vi "Dashboard Main.vi"() -> ()   [LabVIEW 2011]
uses:
  subStates.ctl
  <vilib>/Rock Robotics/WPI/DriverStation/WPI_DriverStationDigitalData.ctl
  <userlib>/_MGI/1D Array/MGI Running Minimum/MGI Running Minimum (SGL).vi
  <userlib>/_MGI/1D Array/MGI Running Maximum/MGI Running Maximum (SGL).vi
  <userlib>/_MGI/1D Array/MGI Running Average/MGI Running Average(SGL).vi
panel:
  in  "Target Overlay":bool=TRUE
  in  "Video Enable":bool=TRUE
  out "Camera Image":T1(plugin-control)
  in  "Info Tabz":enum32{"Comp", "Debug", "UberDebug", "Stats"}(tab)
  out "Shooter Bias":dbl(slide) caption="SHOOTER BIAS" scale=-0.2..0.2
  out "TURRET SAFETY":bool
  out "TURRET LIMIT":bool
  out "GEAR":bool
  out "TRACKING":bool
  out "HOLD":bool
  out "VLAD":bool
  out "Shooter Speed Comp":dbl(slide) caption="SHOOTER SPEED" scale=0.0..100.0
  out "Rest of Custom Data":string
  out "Solenoid Output":bool[](array[boolean])
  out "Robot IP Address":string
  out "8 -- Battery":sgl(graph)
  out "Analog Input":sgl[](array[slide]) scale=0.0..5.0
  out "PWM":cluster{u8, u8}[](array[slide])=[{0, 157}, {0, 157}, {0, 157}, {0, 157}, {0, 157}, {0, 157}, {0, 157}, {0, 157}, {0, 157}, {0, 169}] scale=1.0..255.0
  out "GPIO Output Enable":bool[](array[boolean])
  out "GPIO State":bool[](array[boolean])
  out "Relay":cluster{"Forward":bool[], "Reverse":bool[]}
  out "Shooter Speed":dbl(slide) scale=0.0..100.0 scale format="%#.2g%f"
  out "Safety":bool
  out "Turret Distance":dbl caption="Distance" format="%#_3g"
  out "Turret Rate":dbl caption="Rate" format="%#_3g"
  out "Right Distance":dbl caption="Distance" format="%#_3g"
  out "Right Rate":dbl caption="Rate" format="%#_3g"
  out "Left Distance":dbl caption="Distance" format="%#_3g"
  out "Left Rate":dbl caption="Rate" format="%#_3g"
  out "Angle":dbl(knob) scale=-45.0..45.0 scale format="%#_3g"
  out "Ang. Rate":dbl(knob) scale=-45.0..45.0 scale format="%#_3g"
  out "Lower Belts":T2
  out "Upper Belts":T2
  out "Shooter":T2
  out "Turret":T2
  out "Drive":T2
  out "CPU Usage":dbl(knob) scale=0.0..100.0
  out "RAM Available":u32
  out "Average":dbl
  out "Low":sgl
  out "High":sgl
  out "Battery Voltage":sgl(slide) scale=0.0..15.0
  out "Main IPS":dbl
  out "Vision IPS":dbl
  out "IPS":cluster{dbl, dbl}(knob)={0.0, 16.607957775505273} scale=0.0..60.0
  out "Main mSPI":u32
  out "Vision mSPI":u32
  out "Dashboard Datatype Warning":string="Warning: The Dashboard Datatype used by the robot project and this dashboard do not match.\nSee diagram for more details."
  out "Image Error Message":string="Timeout in Camera Communications"
  # "Solenoid #1"
  # "1"
  # "8"
  # "Communications"
  # "Analog #1"
  # "1"
  # "7"
  # "Digital #1"
  # "1"
  # "10"
  # "1"
  # "14"
  # "1"
  # "8"
  # "Robot States"
  # "Drive Encoders"
  # "Left"
  # "Right"
  # "Turret"
  # "Robot Angle"
  # "Code Speed"
  # "Robot Battery"
  # "cRIO Performance"
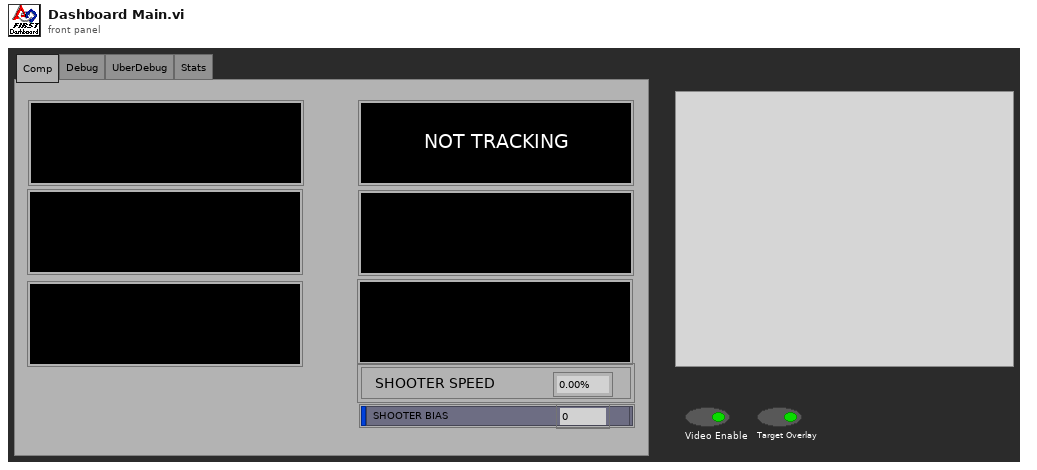
[diagram p1: front panel]
types:
  T1 = typedef "IMAQ Image.ctl" = refnum<image>
  T2 = typedef "subStates.ctl" = enum16{"null", "wait", "driver control", "auto", "manual override", "autoDrive", "hold position", "end"}
  T3 = cluster{"doubles":cluster{"Shooter Speed":dbl, "Turret Rate":dbl, "Turret Distance":dbl, "Right Distance":dbl, "Right Rate":dbl, "Left Rate":dbl, "Left Distance":dbl, "Ang. Rate":dbl, "Angle":dbl, "Shooter Bias":dbl}, "substates":cluster{"Shooter":T2, "Upper Belts":T2, "Lower Belts":T2, "Turret ":T2, "Drive":T2}, "bools":cluster{"VLAD Balanced":bool, "Safety":bool, "Turret Limit":bool}, "Performance":cluster{"CPU Usage":dbl, "RAM Available":u32, "Vision mSPI":u32, "Main mSPI":u32}, "Target Info":cluster{"Left":i32, "Top":i32, "Right":i32, "Bottom":i32}}
  T4 = typedef "WPI_DriverStationDigitalData.ctl" = cluster{"Relay Fwd":u8, "Relay Rev":u8, "GPIO":u16, "GPIO_OE":u16, "PWM":cluster{"PWM[0]":u8, "PWM[1]":u8, "PWM[2]":u8, "PWM[3]":u8, "PWM[4]":u8, "PWM[5]":u8, "PWM[6]":u8, "PWM[7]":u8, "PWM[8]":u8, "PWM[9]":u8}}
  T5 = cluster{cluster{"AnalogModule[0]":cluster{"Channel[0]":sgl, "Channel[1]":sgl, "Channel[2]":sgl, "Channel[3]":sgl, "Channel[4]":sgl, "Channel[5]":sgl, "Channel[6]":sgl, "Channel[7]":sgl}, "AnalogModule[1]":cluster{"Channel[0]":sgl, "Channel[1]":sgl, "Channel[2]":sgl, "Channel[3]":sgl, "Channel[4]":sgl, "Channel[5]":sgl, "Channel[6]":sgl, "Channel[7]":sgl}}, cluster{"DigitalModule[0]":T4, "DigitalModule[1]":T4}, "Solenoid":u8}
  T6 = typedef "Image Type" = u32
  T7 = cluster{"Left":i32, "Top":i32, "Right":i32, "Bottom":i32}
  T8 = cluster{"Competition mode":bool, "Robot Link":bool, "Autonomous":bool, "Enabled":bool, "E-Stop":bool}
  T9 = cluster{"Left":bool, "Top":bool, "Right":bool, "Bottom":bool}
  T10 = cluster{"AnalogModule[0]":cluster{"Channel[0]":sgl, "Channel[1]":sgl, "Channel[2]":sgl, "Channel[3]":sgl, "Channel[4]":sgl, "Channel[5]":sgl, "Channel[6]":sgl, "Channel[7]":sgl}, "AnalogModule[1]":cluster{"Channel[0]":sgl, "Channel[1]":sgl, "Channel[2]":sgl, "Channel[3]":sgl, "Channel[4]":sgl, "Channel[5]":sgl, "Channel[6]":sgl, "Channel[7]":sgl}}
  T11 = cluster{"DigitalModule[0]":T4, "DigitalModule[1]":T4}
  T12 = cluster{"Channel[0]":sgl, "Channel[1]":sgl, "Channel[2]":sgl, "Channel[3]":sgl, "Channel[4]":sgl, "Channel[5]":sgl, "Channel[6]":sgl, "Channel[7]":sgl}[]
  T13 = cluster{"Channel[0]":sgl, "Channel[1]":sgl, "Channel[2]":sgl, "Channel[3]":sgl, "Channel[4]":sgl, "Channel[5]":sgl, "Channel[6]":sgl, "Channel[7]":sgl}
  T14 = typedef "LVRectTypeDef.ctl" = cluster{"left":i16, "top":i16, "right":i16, "bottom":i16}
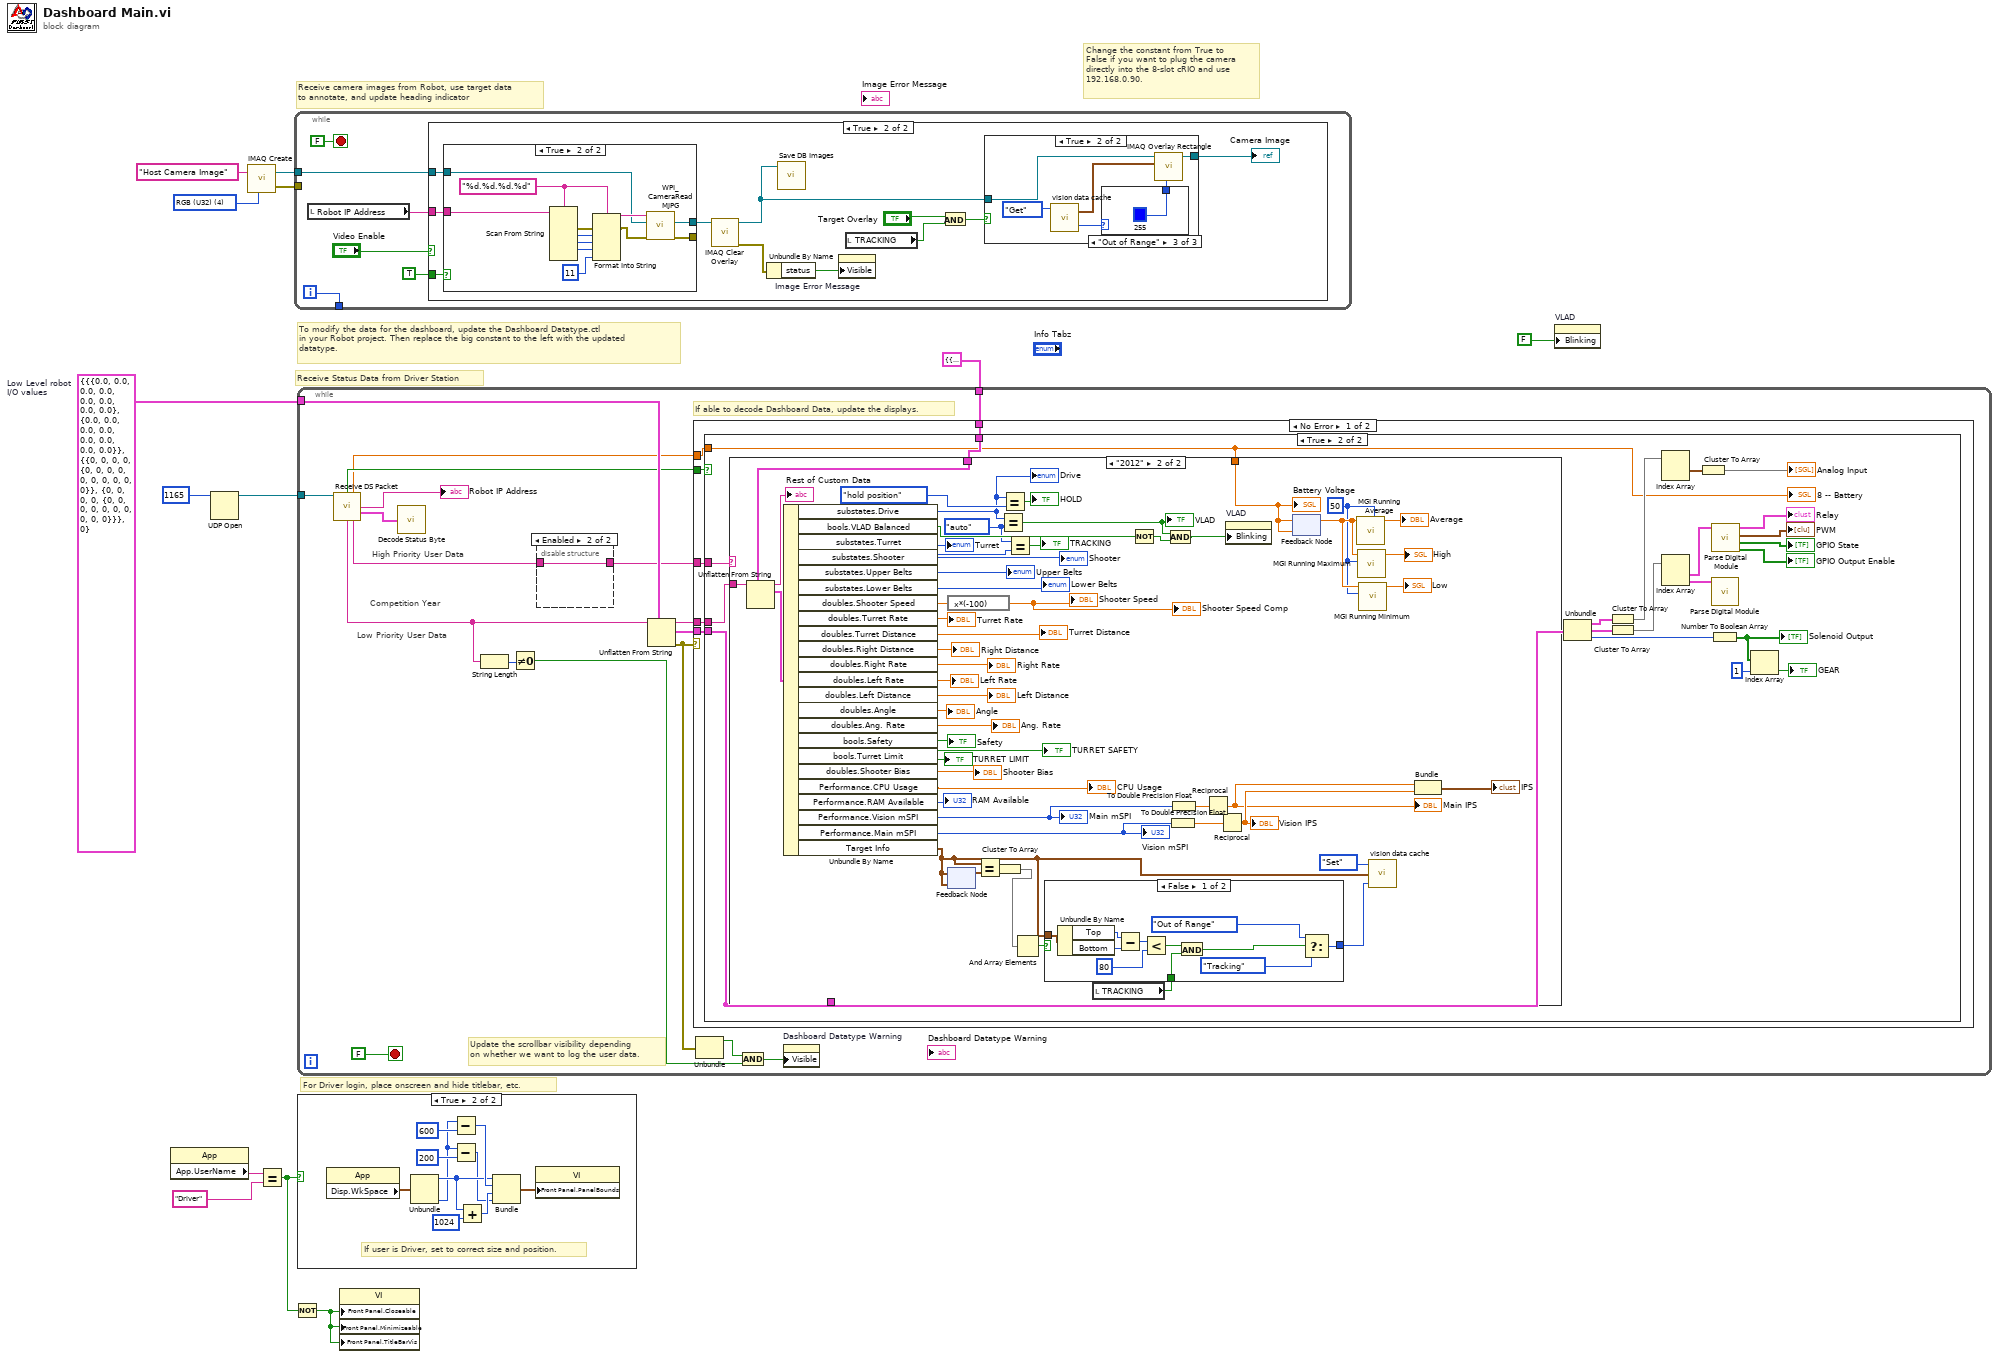
[diagram p0: block diagram]
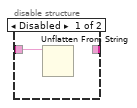
[diagram p3: hidden frame]
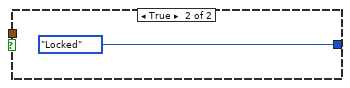
[diagram p6: hidden frame]
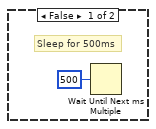
[diagram p8: hidden frame]
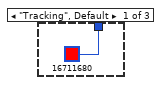
[diagram p10: hidden frame]
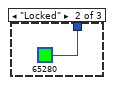
[diagram p11: hidden frame]
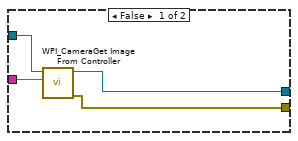
[diagram p12: hidden frame]
diagram:
  w5 = T5 {{"AnalogModule[0]"={"Channel[0]"=0.0, "Channel[1]"=0.0, "Channel[2]"=0.0, "Channel[3]"=0.0, "Channel[4]"=0.0, "Channel[5]"=0.0, "Channel[6]"=0.0, "Channel[7]"=0.0}, "AnalogModule[1]"={"Channel[0]"=0.0, "Channel[1]"=0.0, "Channel[2]"=0.0, "Channel[3]"=0.0, "Channel[4]"=0.0, "Channel[5]"=0.0, "Channel[6]"=0.0, "Channel[7]"=0.0}}, {"DigitalModule[0]"={"Relay Fwd"=0, "Relay Rev"=0, "GPIO"=0, "GPIO_OE"=0, "PWM"={"PWM[0]"=0, "PWM[1]"=0, "PWM[2]"=0, "PWM[3]"=0, "PWM[4]"=0, "PWM[5]"=0, "PWM[6]"=0, "PWM[7]"=0, "PWM[8]"=0, "PWM[9]"=0}}, "DigitalModule[1]"={"Relay Fwd"=0, "Relay Rev"=0, "GPIO"=0, "GPIO_OE"=0, "PWM"={"PWM[0]"=0, "PWM[1]"=0, "PWM[2]"=0, "PWM[3]"=0, "PWM[4]"=0, "PWM[5]"=0, "PWM[6]"=0, "PWM[7]"=0, "PWM[8]"=0, "PWM[9]"=0}}}, "Solenoid"=0}  # Low Level robot I/O values
  w13 = T6 4 items=["Grayscale (U8)", "Grayscale (I16)", "Grayscale (SGL)", "Complex (CSG)", "RGB (U32)", "HSL (U32)", "RGB (U64)"] ("Image Type")
  # "Change the constant from True to\nFalse if you want to plug the camera\ndirectly into the 8-slot cRIO and use\n192.168.0.90."
  # "For Driver login, place onscreen and hide titlebar, etc."
  # "To modify the data for the dashboard, update the Dashboard Datatype.ctl\nin your Robot project. Then replace the big constant to the left with the updated\ndatatype."
  # "Receive Status Data from Driver Station"
  # "Receive camera images from Robot, use target data\nto annotate, and update heading indicator"
  n1 = property class="App"() -> ("App.UserName"=w8:string)  [unwired: 2 in, 2 out]
  n2 = UDP Open(11:u16 1165 ("port")) -> (port=w3:refnum<k16>)  [unwired: 2 in, 4 out]
  n3 = call "IMAQ Create"("Image Name"="Host Camera Image", "Image Type"=w13) -> ("New Image"=w11:T1, "error out"=w10:errorcluster)  [unwired: 2 in, 1 out]
  n4 = Equal?(x=w8, y="Driver") -> (x = y?=w7:bool)
  n5 = Not(x=w7) -> (.not. x?=w6:bool)
  n6 = while {
    tunnel: w11 -> [w17]
    tunnel: w10 -> [_]
    tunnel: [w14] -> _
    i -> [w14]
    stop <- FALSE stop-if-true
    n7 = local read "Robot IP Address"() -> (w18:string)
    n8 = case shown="True" "Video Enable" {
      tunnel: w18 -> [_ w31]
      tunnel: w17 -> [_ w30]
      tunnel: TRUE -> [_ w26]
      frame False {
        # "Sleep for 500ms"
        n9 = Wait Until Next ms Multiple(millisecond multiple=u32 500) -> ()  [unwired: 1 out]
      }
      frame True {
        n10 = case shown="True" w26 {
          tunnel: w30 -> [w44 w51]
          tunnel: [w42 w49] -> _
          tunnel: [w43 w50] -> w27
          tunnel: w31 -> [w45 w54]
          frame False {
            n11 = call <vilib>:"WPI_CameraGet Image From Controller.vi"("Controller Address"=w45, "Image"=w44) -> ("error out"=w42:errorcluster, "Image Out"=w43:T1)  [unwired: 2 in, 6 out]
          }
          frame True {
            w46 = "%d.%d.%d.%d" ("format string")
            n12 = Scan From String(format string=w46, input string=w54) -> (error out=w53:errorcluster, output 1=w55:i32, output 2=w56:i32, output 3=w57:i32)  [unwired: 2 in, 7 out]
            n13 = Format Into String(format string=w46, error in=w53, w55, w56, w57, 11 ("IP Suffix:")) -> (resulting string=w52:string, error out=w48:errorcluster)  [unwired: 1 in]
            n14 = call <vilib>:"WPI_CameraRead MJPG.vi"("error in"=w48, "Image"=w51, "address"=w52) -> ("error out"=w49:errorcluster, "Image Out"=w50:T1)  [unwired: 7 in]
          }
        }
        n15 = call "IMAQ Clear Overlay"("Image"=w27) -> ("error out"=w28:errorcluster, "Image Out"=w25:T1)  [unwired: 2 in, 7 out]
        n16 = Unbundle By Name(w28) -> ("status"=w29:bool)
        n17 = call "Save DB Images.vi"("Image"=w25) -> ()  [unwired: 2 in, 1 out]
        n18 = property on="Image Error Message" class="Str"("Visible"=w29) -> ()  [unwired: 2 in, 2 out]
        n19 = local read "TRACKING"() -> (w22:bool)
        n20 = And(x="Target Overlay", y=w22) -> (x .and. y?=w21:bool)
        n21 = case shown="True" w21 {
          tunnel: w25 -> [w32 w38]
          tunnel: [w32 w35] -> w24
          frame False {
          }
          frame True {
            n22 = call "vision data cache.vi"("Menu (Get)"=enum16{"Get", "Set"}."Get") -> ("State Out"=w34:enum16{"Tracking", "Locked", "Out of Range"}, "Data Output"=w36:T7)  [unwired: 2 in]
            n23 = case shown="\"Out of Range\"" w34 {
              tunnel: [u32 16711680 ("Color") u32 65280 ("Color") u32 255 ("Color")] -> w33
              frame "Tracking", Default {
              }
              frame "Locked" {
              }
              frame "Out of Range" {
              }
            }
            n24 = call "IMAQ Overlay Rectangle"("Color"=w33, "Rectangle"=w36, "Image"=w38) -> ("Image Out"=w35:T1)  [unwired: 3 in, 5 out]
          }
        }
        "Camera Image" <- w24
      }
    }
  }
  n25 = while {
    tunnel: w3 -> [w73]
    tunnel: w5 -> [w72]
    tunnel: T3 {"doubles"={"Shooter Speed"=0.0, "Turret Rate"=0.0, "Turret Distance"=0.0, "Right Distance"=0.0, "Right Rate"=0.0, "Left Rate"=0.0, "Left Distance"=0.0, "Ang. Rate"=0.0, "Angle"=0.0, "Shooter Bias"=0.0}, "substates"={"Shooter"=enum."null", "Upper Belts"=enum."null", "Lower Belts"=enum."null", "Turret "=enum."null", "Drive"=enum."null"}, "bools"={"VLAD Balanced"=FALSE, "Safety"=FALSE, "Turret Limit"=FALSE}, "Performance"={"CPU Usage"=0.0, "RAM Available"=0, "Vision mSPI"=0, "Main mSPI"=0}, "Target Info"={"Left"=0, "Top"=0, "Right"=0, "Bottom"=0}} ("Custom Dash Data") -> [w59]
    stop <- FALSE stop-if-true
    # "Competition Year"
    # "High Priority User Data"
    # "Low Priority User Data"
    # "Update the scrollbar visibility depending\non whether we want to log the user data."
    # "If able to decode Dashboard Data, update the displays."
    n26 = call "Receive DS Packet.vi"("Recv Socket"=w73) -> ("New Dashboard Data"=w69:bool, "Battery"=w60:sgl, "Robot IP Address"=→"Robot IP Address":string, "Status"=w74:T8, "Low Priority User Data"=w62:string, "High Priority User Data"=w61:string)  [unwired: 1 in, 8 out]
    n27 = call "Decode Status Byte.vi"("Status Byte"=w74) -> ()  [unwired: 2 out]
    n28 = String Length(string=w62) -> (length=w64:i32)
    n29 = Not Equal To 0?(x=w64) -> (x != 0?=w67:bool)
    n30 = disable-structure shown="Enabled" {
      disable-tunnel: w61 -> [w76 w77]
      disable-tunnel: [_ w77] -> w58
      frame Disabled {
        n31 = Unflatten From String(binary string=w76) -> ()  [unwired: 2 in, 5 out]
      }
      frame Enabled {
      }
    }
    n32 = Unflatten From String(type=w72, binary string=w62) -> (rest of the binary string=w65:string, value=w71:T5, error out=w70:errorcluster)  [unwired: 1 in, 2 out]
    n33 = case shown="No Error" w70 {
      tunnel: w71 -> [w83 _]
      tunnel: w69 -> [w82 _]
      tunnel: w65 -> [w79 _]
      tunnel: w60 -> [w81 _]
      tunnel: w58 -> [w80 _]
      tunnel: w59 -> [w78 _]
      frame No Error {
        n34 = case shown="True" w82 {
          tunnel: w83 -> [_ w90]
          tunnel: w81 -> [_ w84]
          tunnel: w80 -> [_ w91]
          tunnel: w79 -> [_ w89]
          tunnel: w78 -> [_ w88]
          frame False {
            # "Don't update if the robot hasn't sent new data"
          }
          frame True {
            n35 = case shown="\"2012\"" w91 {
              tunnel: w90 -> [_ _]
              tunnel: w89 -> [_ w156]
              tunnel: w88 -> [_ w157]
              tunnel: w84 -> [_ w121]
              frame "False", Default {
              }
              frame "2012" {
                w117 = 50 ("Averaging Size")
                w114 = subStates."auto" ("y")
                n36 = Unflatten From String(type=w157, binary string=w156) -> (rest of the binary string=→"Rest of Custom Data":string, value=w155:T3)  [unwired: 1 in, 3 out]
                n37 = Unbundle By Name(w155) -> ("substates.Drive"=w136:T2, "bools.VLAD Balanced"=w139:bool, "substates.Turret"=w113:T2, "substates.Shooter"=→"Shooter":T2, "substates.Upper Belts"=→"Upper Belts":T2, "substates.Lower Belts"=→"Lower Belts":T2, "doubles.Shooter Speed"=w150:dbl, "doubles.Turret Rate"=→"Turret Rate":dbl, "doubles.Turret Distance"=→"Turret Distance":dbl, "doubles.Right Distance"=→"Right Distance":dbl, "doubles.Right Rate"=→"Right Rate":dbl, "doubles.Left Rate"=→"Left Rate":dbl, "doubles.Left Distance"=→"Left Distance":dbl, "doubles.Angle"=→"Angle":dbl, "doubles.Ang. Rate"=→"Ang. Rate":dbl, "bools.Safety"=→"Safety" →"TURRET SAFETY":bool, "bools.Turret Limit"=→"TURRET LIMIT":bool, "doubles.Shooter Bias"=→"Shooter Bias":dbl, "Performance.CPU Usage"=→"CPU Usage":dbl, "Performance.RAM Available"=→"RAM Available":u32, "Performance.Vision mSPI"=w129:u32, "Performance.Main mSPI"=w127:u32, "Target Info"=w107:T7)
                "Drive" <- w136
                "Turret" <- w113
                "Main mSPI" <- w129
                "Vision mSPI" <- w127
                n38 = expression code="x*(-100)"(w150) -> (→"Shooter Speed" →"Shooter Speed Comp":dbl)
                n39 = feedback-in #1(w107) -> ()
                n40 = feedback #1(w107) -> (w111:T7)
                n41 = Equal?(x=w107, y=w111) -> (x = y?=w109:T9)
                n42 = Cluster To Array(cluster=w109) -> (array=w110:bool[])
                n43 = Equal?(x=w136, y=w114) -> (x = y?=w115:bool)
                "VLAD" <- w115
                n44 = Equal?(x=w136, y=subStates."hold position" ("x")) -> (x = y?=→"HOLD":bool)
                n45 = Equal?(x=w114, y=w113) -> (x = y?=→"TRACKING":bool)
                n46 = And Array Elements(Boolean array=w110) -> (logical AND=w106:bool)
                n47 = local read "TRACKING"() -> (w105:bool)
                n48 = case shown="False" w106 {
                  tunnel: [w159 enum16{"Tracking", "Locked", "Out of Range"}."Locked" ("State In")] -> w108
                  tunnel: w107 -> [w168 _]
                  tunnel: w105 -> [w162 _]
                  frame False {
                    n49 = Unbundle By Name(w168) -> ("Top"=w158:i32, "Bottom"=w167:i32)
                    n50 = Subtract(x=w158, y=w167) -> (x-y=w166:i32)
                    n51 = Less?(x=w166, y=80) -> (x < y?=w164:bool)
                    n52 = And(x=w164, y=w162) -> (x .and. y?=w163:bool)
                    n53 = Select(t=enum16{"Tracking", "Locked", "Out of Range"}."Out of Range" ("State In"), s=w163, f=enum16{"Tracking", "Locked", "Out of Range"}."Tracking") -> (s? t:f=w159:enum16{"Tracking", "Locked", "Out of Range"})
                  }
                  frame True {
                  }
                }
                n54 = Not(x=w139) -> (.not. x?=w138:bool)
                n55 = And(x=w115, y=w138) -> (x .and. y?=w140:bool)
                n56 = To Double Precision Float(number=w127) -> (double precision float=w126:dbl)
                n57 = To Double Precision Float(number=w129) -> (double precision float=w128:dbl)
                n58 = Reciprocal(x=w128) -> (1/x=w123:dbl)
                "Main IPS" <- w123
                n59 = Reciprocal(x=w126) -> (1/x=w124:dbl)
                "Vision IPS" <- w124
                n60 = property on="VLAD" class="Bool (strict)"("Blinking"=w140) -> ()  [unwired: 2 in, 2 out]
                n61 = feedback-in #2(w121) -> ()
                n62 = feedback #2(w121) -> (w118:sgl)
                n63 = call-poly <userlib>:"MGI Running Average.vi"("Averaging Size"=w117, "Value"=w118) -> ("Average"=→"Average":dbl)  [unwired: 9 in]
                n64 = call-poly <userlib>:"MGI Running Maximum.vi"("Size"=w117, "Value"=w118) -> ("Maximum"=→"High":sgl)  [unwired: 9 in]
                n65 = call-poly <userlib>:"MGI Running Minimum.vi"("Size"=w117, "Value"=w118) -> ("Minimum"=→"Low":sgl)  [unwired: 9 in]
                n66 = call "vision data cache.vi"("State In"=w108, "Data Input"=w107, "Menu (Get)"=enum16{"Get", "Set"}."Set") -> ()  [unwired: 2 out]
                n67 = Bundle(w123, w124) -> (→"IPS":cluster{dbl, dbl})  [unwired: 1 in]
                "Battery Voltage" <- w121
              }
            }
            n68 = Unbundle(w90) -> (w94:T10, w95:T11, "Solenoid"=w96:u8)
            n69 = Cluster To Array(cluster=w94) -> (array=w104:T12)
            n70 = Cluster To Array(cluster=w95) -> (array=w103:T4[])
            n71 = Index Array(array=w104) -> (element #1=w92:T13)  [unwired: 2 in, 1 out]
            n72 = Index Array(array=w103) -> (element #1=w102:T4, element #2=w97:T4)  [unwired: 2 in]
            n73 = Cluster To Array(cluster=w92) -> (array=→"Analog Input":sgl[])
            n74 = call "Parse Digital Module.vi"("DigitalModule"=w97) -> ()  [unwired: 11 out]
            n75 = Number To Boolean Array(number=w96) -> (Boolean array=w87:bool[])
            "Solenoid Output" <- w87
            n76 = call "Parse Digital Module.vi"("DigitalModule"=w102) -> ("GPIO Output Enable"=→"GPIO Output Enable":bool[], "GPIO State"=→"GPIO State":bool[], "PWM"=→"PWM":cluster{u8, u8}[], "Relay"=→"Relay":cluster{"Forward":bool[], "Reverse":bool[]})  [unwired: 7 out]
            n77 = Index Array(array=w87, index=1) -> (element=→"GEAR":bool)
            "8 -- Battery" <- w84
          }
        }
      }
      frame Error {
        # "Your datatypes don't match. The Dashboard Datatype.ctl in your Robot project\nand the big constant to the left of the loop need to match."
      }
    }
    n78 = Unbundle(w70) -> ("status"=w66:bool)  [unwired: 2 out]
    n79 = And(x=w66, y=w67) -> (x .and. y?=w68:bool)
    n80 = property on="Dashboard Datatype Warning" class="Str"("Visible"=w68) -> ()  [unwired: 2 in, 2 out]
  }
  n81 = case shown="True" w7 {
    frame False {
    }
    frame True {
      # "If user is Driver, set to correct size and position."
      n82 = property class="App"() -> ("Disp.WkSpace"=w179:T14)  [unwired: 2 in, 2 out]
      n83 = Unbundle(w179) -> ("left"=w174:i16, "bottom"=w170:i16)  [unwired: 2 out]
      n84 = Subtract(x=w170, y=600) -> (x-y=w176:i32)
      n85 = Subtract(x=w170, y=200) -> (x-y=w171:i32)
      n86 = Add(x=w174, y=1024) -> (x+y=w175:i32)
      n87 = Bundle("left"=w174, w176, w175, w171) -> (w178:cluster{"left":i16, i32, i32, i32})  [unwired: 1 out]
      n88 = property class="VI"("Front Panel.PanelBounds"=w178) -> ()  [unwired: 2 in, 2 out]
    }
  }
  n89 = property class="VI"("Front Panel.Closeable"=w6, "Front Panel.Minimizeable"=w6, "Front Panel.TitleBarVis"=w6) -> ()  [unwired: 2 in, 2 out]
  n90 = property on="VLAD" class="Bool (strict)"("Blinking"=FALSE) -> ()  [unwired: 2 in, 2 out]
